vi "Target Tracking.vi"() -> (0 "Joystick Y":dbl, 3 "Joystick X":dbl)   [LabVIEW 2019]
uses:
  <vilib>/Rock Robotics/Network Tables/NT Read Number.vi
  Robot Global Data.vi
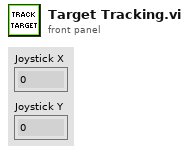
[diagram p1: front panel]
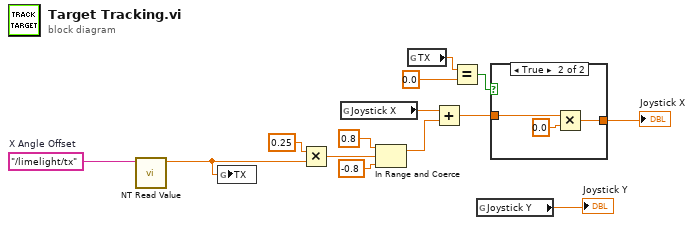
[diagram p0: block diagram]
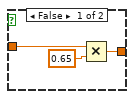
[diagram p2: hidden frame]
diagram:
  w3 = "/limelight/tx"  # X Angle Offset
  n1 = call-poly <vilib>:"NT Read Value.vi"("Name"=w3) -> ("Numeric"=w14:dbl)  [unwired: 9 in, 1 out]
  n2 = global write "Robot Global Data.vi" "TX"(w14) -> ()
  n3 = Multiply(x=0.25 ("y"), y=w14) -> (x*y=w6:dbl)
  n4 = global read "Robot Global Data.vi" "Joystick X"() -> (w4:dbl)
  n5 = In Range and Coerce(upper limit=0.8, x=w6, lower limit=-0.8) -> (coerced(x)=w5:dbl)  [unwired: 1 out]
  n6 = global read "Robot Global Data.vi" "TX"() -> (w12:dbl)
  n7 = Add(x=w4, y=w5) -> (x+y=w10:dbl)
  n8 = Equal?(x=w12, y=0.0) -> (x = y?=w11:bool)
  n9 = global read "Robot Global Data.vi" "Joystick Y"() -> (→"Joystick Y":dbl)
  n10 = case shown="True" w11 {
    tunnel: w10 -> [w16 w20]
    tunnel: [w17 w18] -> w1
    frame False {
      n11 = Multiply(x=w16, y=0.65) -> (x*y=w17:dbl)
    }
    frame True {
      n12 = Multiply(x=w20, y=0.0) -> (x*y=w18:dbl)
    }
  }
  "Joystick X" <- w1
